vi "Enqueue.vi"(7 "Priority (f)":bool, 8 "Error In":errorcluster[](array[cluster]), 9 "Data":variant, 10 "Msg":string, 11 "QueRef":refnum<queue>) -> (0 "Error Out":errorcluster[](array[cluster]), 3 "QueRef":refnum<queue>)   [LabVIEW 2014, in "BusController.lvlib"]
uses:
  BusController.lvlib
  QueueType.ctl
  <userlib>/NIST/NISTErrorLib/NISTErrorLib.lvlib
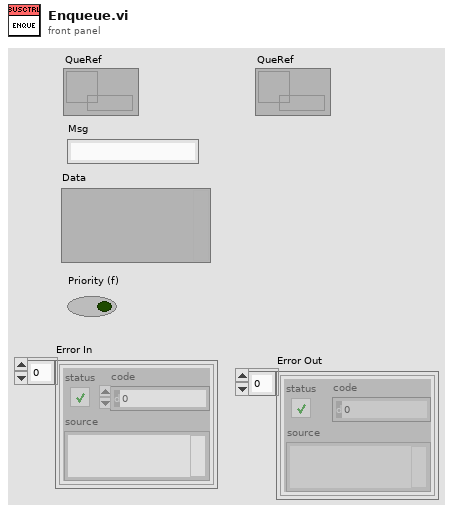
[diagram p1: front panel]
types:
  T1 = typedef "BusController.lvlib/QueueType.ctl" = cluster{"Msg":string, "Data":variant}
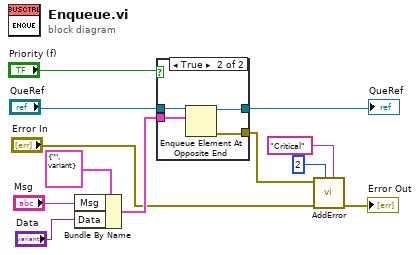
[diagram p0: block diagram]
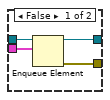
[diagram p2: hidden frame]
diagram:
  n1 = Bundle By Name(cluster=T1 {"Msg"="", "Data"=variant} ("QueueType"), "Msg"="Msg", "Data"="Data") -> (w8:T1)
  n2 = case shown="True" "Priority (f)" {
    tunnel: "QueRef" -> [w16 w20]
    tunnel: w8 -> [w15 w19]
    tunnel: [w14 w18] -> w6
    tunnel: [w13 w17] -> w1
    frame False {
      n3 = Enqueue Element(queue=w16, element=w15) -> (queue out=w13:refnum<queue>, error out=w14:errorcluster)  [unwired: 2 in, 1 out]
    }
    frame True {
      n4 = Enqueue Element At Opposite End(queue=w20, element=w19) -> (queue out=w17:refnum<queue>, error out=w18:errorcluster)  [unwired: 2 in, 1 out]
    }
  }
  "QueRef" <- w1
  n5 = call <userlib>:"AddError.vi"("Severity"="Critical", "Priority"=u8 2, "ErrorArray"="Error In", "error in (no error)"=w6) -> ("ErrorArray"=→"Error Out":errorcluster[])  [unwired: 6 in, 1 out]
